vi "Parse Response Message.vi"(8 "error in":errorcluster, 11 "Newport in":refnum<class "Newport.lvclass">) -> (0 "error out":errorcluster, 3 "Newport out":refnum<class "Newport.lvclass">)   [LabVIEW 2018, in "Newport.lvlib" / "Newport.lvclass"]
uses:
  Newport.lvclass
  Parent/Axis.lvclass
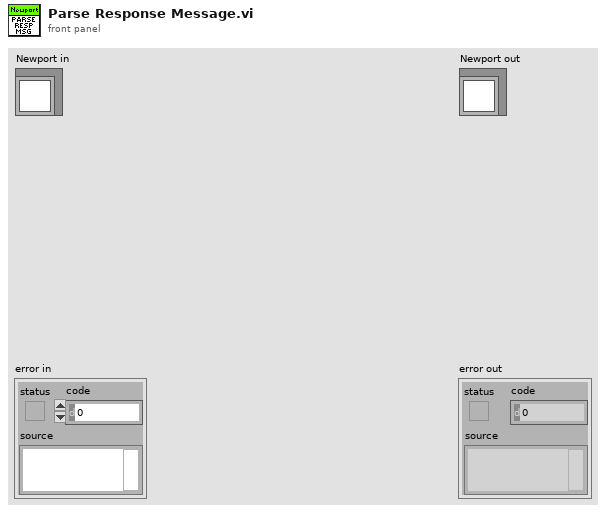
[diagram p1: front panel]
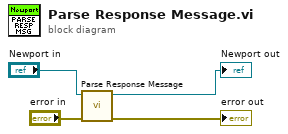
[diagram p0: block diagram]
diagram:
  n1 = call-parent "Parse Response Message.vi"("error in"="error in", "Axis in"="Newport in") -> ("error out"=→"error out":errorcluster, "Axis out"=→"Newport out":refnum<class "Newport.lvclass">)  [unwired: 8 in]
